vi "Example Configuration.vi"() -> ()   [LabVIEW 2010]
uses:
  C:/tf/play/labview/Tinkerforge.dll
  Tinkerforge.dll
panel:
  in  "stop":bool
  in  "uid":string="63oL6P"
  in  "port":i32=4223
  in  "host":string="localhost"
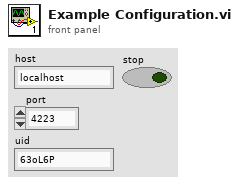
[diagram p1: front panel]
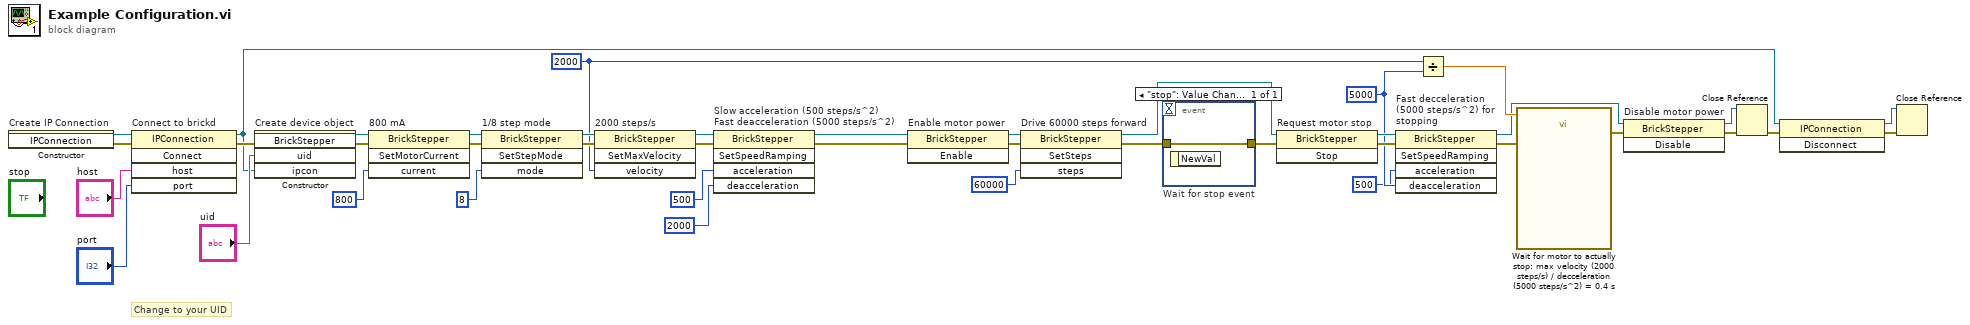
[diagram p0: block diagram]
diagram:
  w5 = 5000 ("deacceleration")
  w4 = 2000 ("velocity")
  # "Change to your UID"
  n1 = constructor on="Create IP Connection" class="IPConnection"() -> (reference out=w41:refnum<k24>, error out=w15:errorcluster)  [unwired: 3 in, 1 out]
  n2 = invoke on="Connect to brickd" class="IPConnection" method="Connect"(reference=w41, error in=w15, "host"="host", "port"="port") -> (reference out=w32:refnum<k24>, error out=w37:errorcluster)  [unwired: 1 in, 3 out]
  n3 = constructor on="Create device object" class="BrickStepper"(error in=w37, "uid"="uid", "ipcon"=w32) -> (reference out=w35:refnum<k24>, error out=w36:errorcluster)  [unwired: 2 in, 3 out]
  n4 = invoke on="800 mA" class="BrickStepper" method="SetMotorCurrent"(reference=w35, error in=w36, "current"=800) -> (reference out=w27:refnum<k24>, error out=w29:errorcluster)  [unwired: 1 in, 2 out]
  n5 = invoke on="1/8 step mode" class="BrickStepper" method="SetStepMode"(reference=w27, error in=w29, "mode"=u8 8) -> (reference out=w26:refnum<k24>, error out=w28:errorcluster)  [unwired: 1 in, 2 out]
  n6 = invoke on="2000 steps/s" class="BrickStepper" method="SetMaxVelocity"(reference=w26, error in=w28, "velocity"=w4) -> (reference out=w23:refnum<k24>, error out=w24:errorcluster)  [unwired: 1 in, 2 out]
  n7 = invoke on="Slow acceleration (500 steps/s^2)\nFast deacceleration (5000 steps/s^2)" class="BrickStepper" method="SetSpeedRamping"(reference=w23, error in=w24, "acceleration"=500, "deacceleration"=2000) -> (reference out=w19:refnum<k24>, error out=w20:errorcluster)  [unwired: 1 in, 3 out]
  n8 = invoke on="Enable motor power" class="BrickStepper" method="Enable"(reference=w19, error in=w20) -> (reference out=w17:refnum<k24>, error out=w18:errorcluster)  [unwired: 1 in, 1 out]
  n9 = invoke on="Drive 60000 steps forward" class="BrickStepper" method="SetSteps"(reference=w17, error in=w18, "steps"=60000) -> (reference out=w10:refnum<k24>, error out=w1:errorcluster)  [unwired: 1 in, 2 out]
  n10 = event "Wait for stop event" shown="[0] \"stop\": Value Change" {
    selector: _ -> [_]
    dyn-events: _ -> [_]
    timeout: _ -> [_]
    tunnel: [w42] -> w2
    tunnel: w1 -> [w42]
    event "stop": Value Change {
      n11 = event-data() -> ()  [unwired: 1 in, 1 out]
    }
  }
  n12 = invoke on="Request motor stop" class="BrickStepper" method="Stop"(reference=w10, error in=w2) -> (reference out=w9:refnum<k24>, error out=w7:errorcluster)  [unwired: 1 in, 1 out]
  n13 = invoke on="Fast decceleration\n(5000 steps/s^2) for\nstopping" class="BrickStepper" method="SetSpeedRamping"(reference=w9, error in=w7, "acceleration"=500, "deacceleration"=w5) -> (reference out=w8:refnum<k24>, error out=w6:errorcluster)  [unwired: 1 in, 3 out]
  n14 = Divide(x=w4, y=w5) -> (x/y=w13:dbl)
  n15 = call "Wait for motor to actually stop: max velocity (2000 steps/s) / decceleration (5000 steps/s^2) = 0.4 s"("error in (no error)"=w6, "Delay Time (s)"=w13) -> ("error out"=w14:errorcluster)  [unwired: 9 in]
  n16 = invoke on="Disable motor power" class="BrickStepper" method="Disable"(reference=w8, error in=w14) -> (reference out=w11:refnum<k24>, error out=w12:errorcluster)  [unwired: 1 in, 1 out]
  n17 = Close Reference(reference=w11, error in (no error)=w12) -> (error out=w34:errorcluster)
  n18 = invoke class="IPConnection" method="Disconnect"(reference=w32, error in=w34) -> (reference out=w31:refnum<k24>, error out=w33:errorcluster)  [unwired: 1 in, 1 out]
  n19 = Close Reference(reference=w31, error in (no error)=w33) -> ()  [unwired: 1 out]
